vi "Generate Tektronix DPO MSO 2000 4000 Series Data.vi"(8 "error in (no error)":errorcluster, 11 "VISA resource name":refnum<visa-resource-name>) -> (0 "error out":errorcluster, 2 "Graph Data":waveform(dbl)[](array[waveform]), 3 "VISA resource name 2":refnum<visa-resource-name>)   [LabVIEW 2016, in "Acquisition.lvlib"]
doc: "Generates sample waveforms according to the signal type in the HW Config input."
uses:
  support/DAQ Drivers/Tektronix DPO MSO 2000 4000 Series/Public/Data/Read (Single Waveform).vi
  Acquisition.lvlib
  support/DAQ Drivers/Tektronix DPO MSO 2000 4000 Series/Tektronix DPO MSO 2000 4000 Series.lvlib
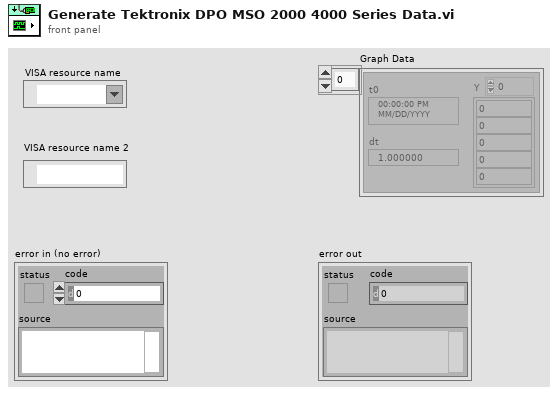
[diagram p1: front panel]
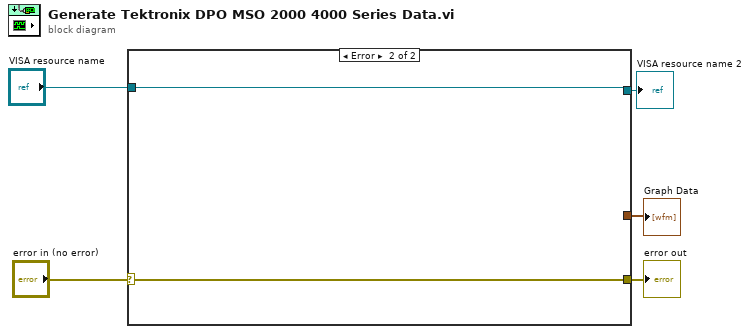
[diagram p0: block diagram]
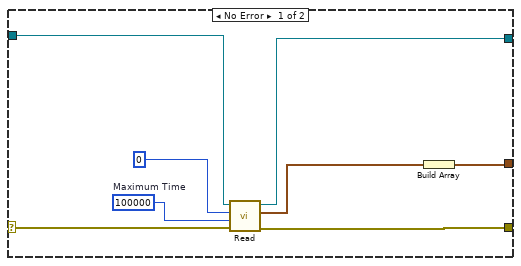
[diagram p2: hidden frame]
diagram:
  n1 = case shown="Error" "error in (no error)" {
    selector: "error in (no error)" -> [w11 w15]
    tunnel: [w10 w15] -> w4
    tunnel: "VISA resource name" -> [w9 w14]
    tunnel: [w6 _] -> w1
    tunnel: [w8 w14] -> w2
    frame No Error {
      w13 = 100000  # Maximum Time
      n2 = call-poly "Read.vi"("error in (no error)"=w11, "Maximum Time (10000ms)"=w13, "Channel (0: Channel 1)"=0, "VISA resource name"=w9) -> ("error out"=w10:errorcluster, "Waveform Graph"=w7:waveform(dbl), "VISA resource name out"=w8:refnum<visa-resource-name>)  [unwired: 5 in]
      n3 = Build Array(w7) -> (w6:waveform(dbl)[])
    }
    frame Error {
    }
  }
  "error out" <- w4
  "Graph Data" <- w1
  "VISA resource name 2" <- w2
